vi "例程24-数据记录文件的读取.vi"() -> ()   [LabVIEW 2016]
panel:
  out "记录":cluster{"温度":dbl, "日期":string, "时间":string}
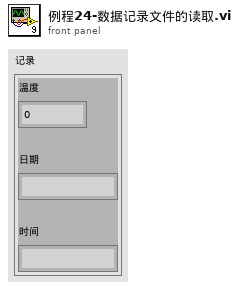
[diagram p1: front panel]
types:
  T1 = enum16{"deny read/write", "deny write-only", "deny none"}
  T2 = enum16{"open", "replace", "create", "open or create", "replace or create", "replace or create with confirmation"}
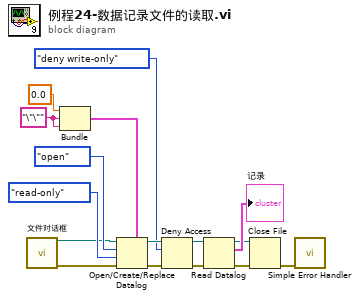
[diagram p0: block diagram]
diagram:
  w8 = "\"\""
  n1 = call "文件对话框"() -> ("selected path"=w14:path, "error out"=w13:errorcluster)  [unwired: 12 in, 2 out]
  n2 = Bundle(0.0, w8, w8) -> (w7:cluster{dbl, string, string})  [unwired: 1 in]
  n3 = Open/Create/Replace Datalog(5:w7, 8:w13, 9:enum16{"read/write", "read-only", "write-only"}."read-only" ("权限(0:read/write)"), 10:T2."open" ("操作(0:open)"), 11:w14) -> (0:w11:errorcluster, 3:w12:refnum<k1>)  [unwired: 1 in, 1 out]
  n4 = Deny Access(4:w11, 6:T1."deny write-only" ("限制模式(0:读/写限制)"), 7:w12) -> (0:w6:errorcluster, 3:w5:refnum<k1>)
  n5 = Read Datalog(4:w6, 7:w5) -> (0:w2:errorcluster, 2:→"记录":cluster{dbl, string, string}, 3:w3:refnum<k1>)  [unwired: 1 in]
  n6 = Close File(refnum=w3, error in=w2) -> (error out=w1:errorcluster)  [unwired: 1 out]
  n7 = call <vilib>:"Simple Error Handler.vi"("error in (no error)"=w1) -> ()  [unwired: 4 in, 5 out]
